vi "DetectCollisionSmoother.vi"(0 "Goal":dbl[](array[numeric]), 4 "Initial State":dbl[](array[numeric]), 6 "enemy_robots":T1[](array[typedef]), 7 "Robot in":T1={"id"=0, "function"=enum."Attacker", "x"=0.0, "y"=0.0, "orientation"=0.0, "v_tangent"=0.0, "v_normal"=0.0, "v_ang"=0.0, "kick_x"=0.0, "kick_z"=0.0, "dribble"=FALSE, "Timestamp"=timestamp(0 s since 1904-01-01), "estimatives"={"est_v_tangent"=0.0, "est_v_normal"=0.0, "est_vx"=0.0, "est_vy"=0.0, "Pos Robot Est"=[]}, "dest_x_kick"=0.0, "dest_y_kick"=0.0, "Gap Coord"=[], "States"=enum."Pass", "Path "=[], "Path  Smooth"=[], "Dest"=[], "vx_desired"=0.0, "vy_desired"=0.0}, 8 "SegmentPointB":dbl[](array[numeric]), 9 "SegmentPointA":dbl[](array[numeric]), 10 "ball":dbl[](array[numeric])) -> (3 "Is there colision?":bool)   [LabVIEW 2020]
uses:
  Vision_class/Old vision/Controls/AI Robot.ctl
  Vision_class/Old vision/Controls/Functions Enum.ctl
  Vision_class/Old vision/Controls/AttackerStates.ctl
  Vision_class/Old vision/Controls/PathDests.ctl
  Vision_class/Old vision/Controls/PathDest.ctl
panel:
  in  "our_robots":T1[](array[typedef])
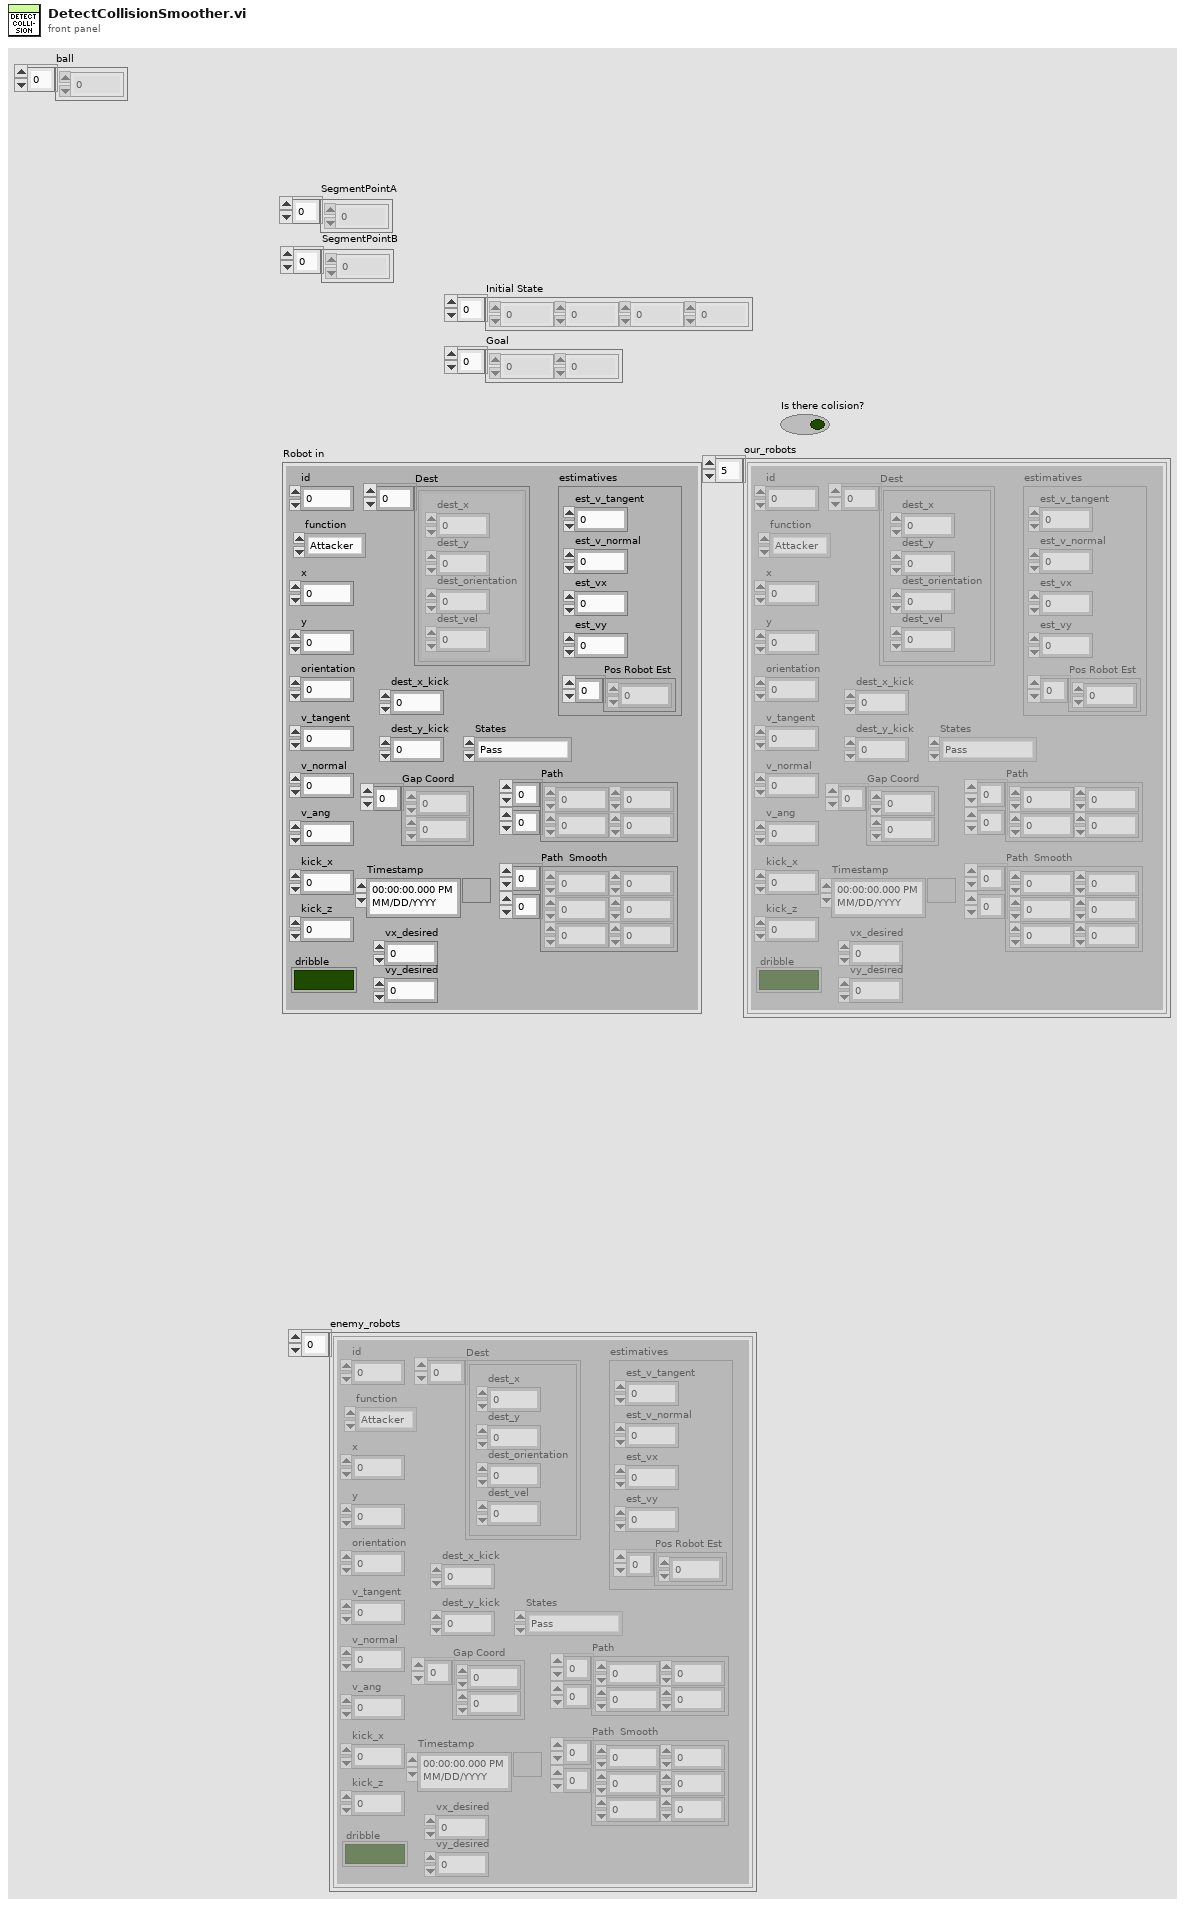
[diagram p1: front panel]
types:
  T1 = typedef "AI Robot.ctl" = cluster{"id":u32, "function":T2, "x":dbl, "y":dbl, "orientation":dbl, "v_tangent":dbl, "v_normal":dbl, "v_ang":dbl, "kick_x":dbl, "kick_z":dbl, "dribble":bool, "Timestamp":timestamp, "estimatives":cluster{"est_v_tangent":dbl, "est_v_normal":dbl, "est_vx":dbl, "est_vy":dbl, "Pos Robot Est":dbl[]}, "dest_x_kick":dbl, "dest_y_kick":dbl, "Gap Coord":dbl[], "States":T3, "Path ":dbl[][], "Path  Smooth":dbl[][], "Dest":T4, "vx_desired":dbl, "vy_desired":dbl}
  T2 = typedef "Functions Enum.ctl" = enum16{"2nd Striker", "Attacker", "Goalie", "Defender", "Striker", "Goto 0", "Dummy", "Kicker", "ZigZag 0", "ZigZag 1", "ZigZag 2", "ZigZag 3", "ZigZag 4", "ZigZag 5", "ZigZag 6", "ZigZag 7", "ZigZag 8", ""}
  T3 = typedef "AttackerStates.ctl" = enum16{"Pass", "GoToTangent", "BallGetting", "GoToKick", ""}
  T4 = typedef "PathDests.ctl" = T5[]
  T5 = typedef "PathDest.ctl" = cluster{"dest_x":dbl, "dest_y":dbl, "dest_orientation":dbl, "dest_vel":dbl}
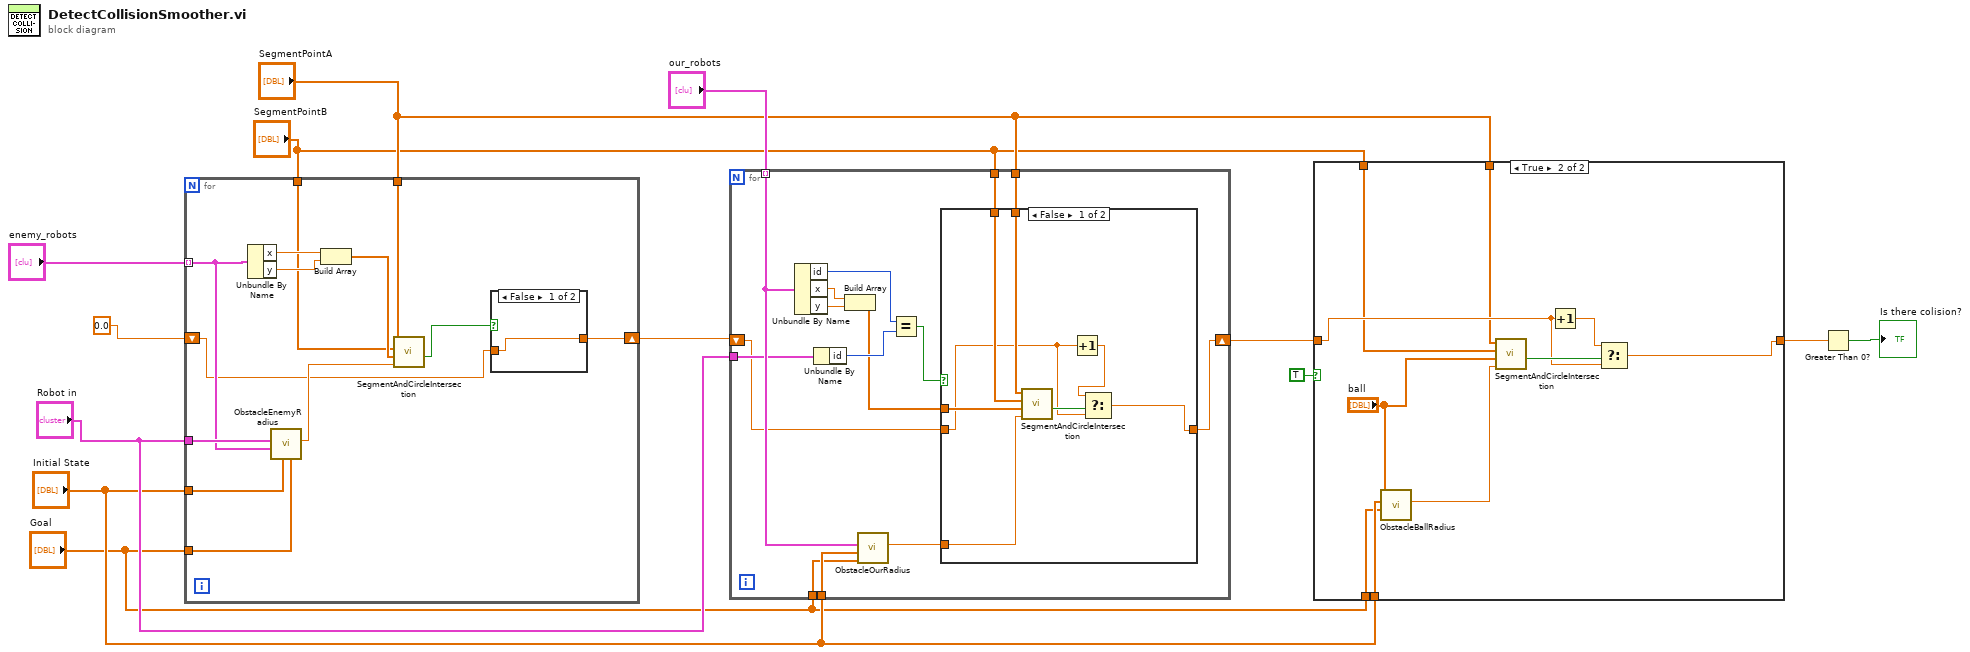
[diagram p0: block diagram]
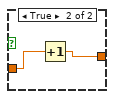
[diagram p4: hidden frame]
diagram:
  n1 = for {
    tunnel: "enemy_robots" -> [w20] mode=indexing
    tunnel: "Initial State" -> [w23]
    tunnel: "Goal" -> [w22]
    tunnel: "Robot in" -> [w21]
    tunnel: "SegmentPointA" -> [w18]
    tunnel: "SegmentPointB" -> [w17]
    shift-right: [w14] -> w9
    shift-left: 0.0 -> [w15]
    n2 = Unbundle By Name(w20) -> ("x"=w26:dbl, "y"=w25:dbl)
    n3 = call "ObstacleEnemyRadius.vi"("Goal"=w22, "Initial State"=w23, "Robot enemy"=w20, "Robot in"=w21) -> ("obstacle enemy radius"=w19:dbl)  [unwired: 7 in]
    n4 = Build Array(w26, w25) -> (w24:dbl[])
    n5 = call "SegmentAndCircleIntersection.vi"("CircleRadius"=w19, "CircleCenter"=w24, "SegmentPointB"=w17, "SegmentPointA"=w18) -> ("DoTheyIntersect?"=w16:bool)  [unwired: 7 in]
    n6 = case shown="False" w16 {
      tunnel: w15 -> [w27 w29]
      tunnel: [w27 w28] -> w14
      frame False {
      }
      frame True {
        n7 = Increment(x=w29) -> (x+1=w28:dbl)
      }
    }
  }
  n8 = for {
    tunnel: "our_robots" -> [w44] mode=indexing
    shift-right: [w37] -> w5
    shift-left: w9 -> [w36]
    tunnel: "Initial State" -> [w43]
    tunnel: "Goal" -> [w42]
    tunnel: "Robot in" -> [w41]
    tunnel: "SegmentPointA" -> [w34]
    tunnel: "SegmentPointB" -> [w33]
    n9 = Unbundle By Name(w44) -> ("id"=w40:u32, "x"=w32:dbl, "y"=w31:dbl)
    n10 = Unbundle By Name(w41) -> ("id"=w39:u32)
    n11 = Build Array(w32, w31) -> (w30:dbl[])
    n12 = call "ObstacleOurRadius.vi"("Goal"=w42, "Initial State"=w43, "other robot"=w44) -> ("obstacle enemy radius"=w35:dbl)  [unwired: 8 in]
    n13 = Equal?(x=w40, y=w39) -> (x = y?=w38:bool)
    n14 = case shown="False" w38 {
      tunnel: [w46 w53] -> w37
      tunnel: w36 -> [w45 w53]
      tunnel: w35 -> [w52 _]
      tunnel: w34 -> [w51 _]
      tunnel: w33 -> [w50 _]
      tunnel: w30 -> [w49 _]
      frame False {
        n15 = call "SegmentAndCircleIntersection.vi"("CircleRadius"=w52, "CircleCenter"=w49, "SegmentPointB"=w50, "SegmentPointA"=w51) -> ("DoTheyIntersect?"=w48:bool)  [unwired: 7 in]
        n16 = Increment(x=w45) -> (x+1=w47:dbl)
        n17 = Select(t=w47, s=w48, f=w45) -> (s? t:f=w46:dbl)
      }
      frame True {
      }
    }
  }
  n18 = case shown="True" TRUE {
    tunnel: [w54 w58] -> w6
    tunnel: w5 -> [w54 w59]
    tunnel: "Initial State" -> [_ w64]
    tunnel: "Goal" -> [_ w63]
    tunnel: "SegmentPointA" -> [_ w57]
    tunnel: "SegmentPointB" -> [_ w56]
    frame False {
    }
    frame True {
      n19 = call "ObstacleBallRadius.vi"("Goal"=w63, "Initial State"=w64, "ball"="ball") -> ("obstacle enemy radius"=w62:dbl)  [unwired: 8 in]
      n20 = call "SegmentAndCircleIntersection.vi"("CircleRadius"=w62, "CircleCenter"="ball", "SegmentPointB"=w56, "SegmentPointA"=w57) -> ("DoTheyIntersect?"=w61:bool)  [unwired: 7 in]
      n21 = Increment(x=w59) -> (x+1=w60:dbl)
      n22 = Select(t=w60, s=w61, f=w59) -> (s? t:f=w58:dbl)
    }
  }
  n23 = Greater Than 0?(x=w6) -> (x > 0?=→"Is there colision?":bool)
